vi "String to Control loop cluster.vi"(11 "Control Loop Details":string="EXCT:TYPE:Unipolar:MAG:10.00:EXCT:NICK:MB1.T1:LOOP:AUX:None:PSET:1.0:HTR:None:ISET:1.0:HAUT:Manual:HSET:0.0:PIDT:Manual:DSET:1.0:TSET:0K:LVL:MB1.T1:LOOP:MAN:HVER:0:FVER:20.6:SERL:102750119:MAN:CAL:OFFS:0.0000:COLD:1.0000:INT:Linear:SCAL:1.0000:FILE:RP5.DAT:HOTL:1023.1500:CAL:TYPE:PTC:SIG:VOLT:1405.9mV:CURR:10µA:TEMP:1023.15K:POWR:14.059µW:RES:140590?:SLOP:137.409?/K:FLOW:NOT_FOUND:SIG:TEMP\n") -> (3 "Control Loop":T1)   [LabVIEW 2015, in "Mercury iXX.lvlib" / "Control Loop.lvlib"]
uses:
  Control Loop.lvlib
  Temperature/Controls/Loop Cluster.ctl
  Temperature.lvlib
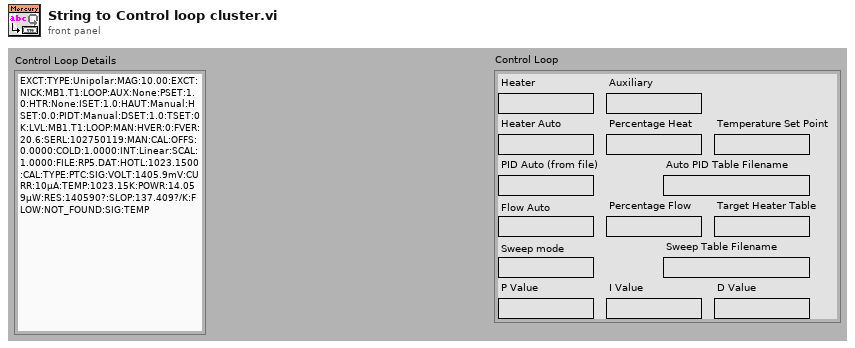
[diagram p1: front panel]
types:
  T1 = typedef "Mercury iXX.lvlib/Temperature.lvlib/Loop Cluster.ctl" = cluster{"Heater":string, "Auxiliary":string, "Heater Auto":string, "Percentage Heat":string, "Temperature Set Point":string, "PID Auto (from file)":string, "P Value":string, "I Value":string, "D Value":string, "Auto PID Table Filename":string, "Flow Auto":string, "Target Heater Table":string, "Sweep mode":string, "Sweep Table Filename":string, "Percentage Flow":string}
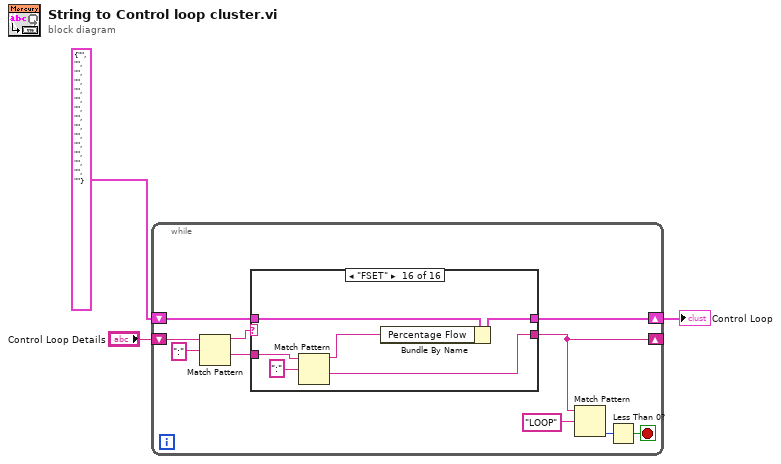
[diagram p0: block diagram]
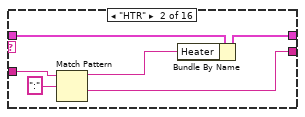
[diagram p3: hidden frame]
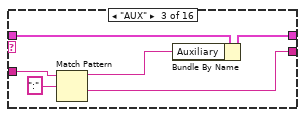
[diagram p4: hidden frame]
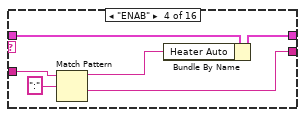
[diagram p5: hidden frame]
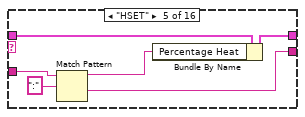
[diagram p6: hidden frame]
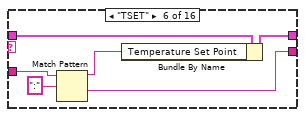
[diagram p7: hidden frame]
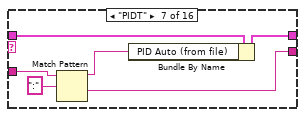
[diagram p8: hidden frame]
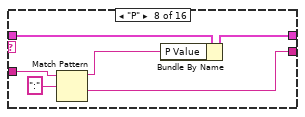
[diagram p9: hidden frame]
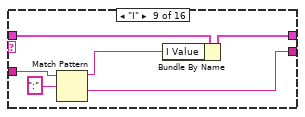
[diagram p10: hidden frame]
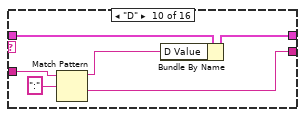
[diagram p11: hidden frame]
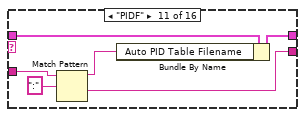
[diagram p12: hidden frame]
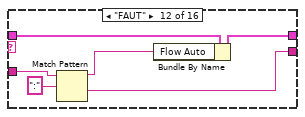
[diagram p13: hidden frame]
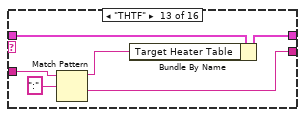
[diagram p14: hidden frame]
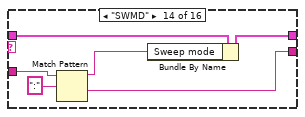
[diagram p15: hidden frame]
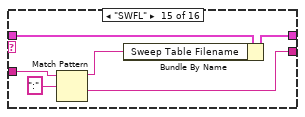
[diagram p16: hidden frame]
diagram:
  n1 = while {
    shift-right: [w6] -> w2
    shift-left: T1 {"Heater"="", "Auxiliary"="", "Heater Auto"="", "Percentage Heat"="", "Temperature Set Point"="", "PID Auto (from file)"="", "P Value"="", "I Value"="", "D Value"="", "Auto PID Table Filename"="", "Flow Auto"="", "Target Heater Table"="", "Sweep mode"="", "Sweep Table Filename"="", "Percentage Flow"=""} ("Control Loop") -> [w7]
    shift-right: [w4] -> _
    shift-left: "Control Loop Details" -> [w12]
    stop <- w9 stop-if-true
    n2 = Match Pattern(string=w12, regular expression=":") -> (before substring=w11:string, after substring=w5:string)  [unwired: 3 out]
    n3 = case shown="\"FSET\"" w11 {
      tunnel: w7 -> [w15 w17 w23 w29 w35 w41 w47 w53 w59 w65 w71 w77 w83 w89 w95 w101]
      tunnel: [w15 w18 w24 w30 w36 w42 w48 w54 w60 w66 w72 w78 w84 w90 w96 w102] -> w6
      tunnel: [w14 w19 w25 w31 w37 w43 w49 w55 w61 w67 w73 w79 w85 w91 w97 w103] -> w4
      tunnel: w5 -> [w14 w20 w26 w32 w38 w44 w50 w56 w62 w68 w74 w80 w86 w92 w98 w104]
      frame "", Default {
      }
      frame "HTR" {
        n4 = Match Pattern(string=w20, regular expression=":") -> (before substring=w16:string, after substring=w19:string)  [unwired: 3 out]
        n5 = Bundle By Name(cluster=w17, "Heater"=w16) -> (w18:T1)
      }
      frame "AUX" {
        n6 = Match Pattern(string=w26, regular expression=":") -> (before substring=w22:string, after substring=w25:string)  [unwired: 3 out]
        n7 = Bundle By Name(cluster=w23, "Auxiliary"=w22) -> (w24:T1)
      }
      frame "ENAB" {
        n8 = Match Pattern(string=w32, regular expression=":") -> (before substring=w28:string, after substring=w31:string)  [unwired: 3 out]
        n9 = Bundle By Name(cluster=w29, "Heater Auto"=w28) -> (w30:T1)
      }
      frame "HSET" {
        n10 = Match Pattern(string=w38, regular expression=":") -> (before substring=w34:string, after substring=w37:string)  [unwired: 3 out]
        n11 = Bundle By Name(cluster=w35, "Percentage Heat"=w34) -> (w36:T1)
      }
      frame "TSET" {
        n12 = Match Pattern(string=w44, regular expression=":") -> (before substring=w40:string, after substring=w43:string)  [unwired: 3 out]
        n13 = Bundle By Name(cluster=w41, "Temperature Set Point"=w40) -> (w42:T1)
      }
      frame "PIDT" {
        n14 = Match Pattern(string=w50, regular expression=":") -> (before substring=w46:string, after substring=w49:string)  [unwired: 3 out]
        n15 = Bundle By Name(cluster=w47, "PID Auto (from file)"=w46) -> (w48:T1)
      }
      frame "P" {
        n16 = Match Pattern(string=w56, regular expression=":") -> (before substring=w52:string, after substring=w55:string)  [unwired: 3 out]
        n17 = Bundle By Name(cluster=w53, "P Value"=w52) -> (w54:T1)
      }
      frame "I" {
        n18 = Match Pattern(string=w62, regular expression=":") -> (before substring=w58:string, after substring=w61:string)  [unwired: 3 out]
        n19 = Bundle By Name(cluster=w59, "I Value"=w58) -> (w60:T1)
      }
      frame "D" {
        n20 = Match Pattern(string=w68, regular expression=":") -> (before substring=w64:string, after substring=w67:string)  [unwired: 3 out]
        n21 = Bundle By Name(cluster=w65, "D Value"=w64) -> (w66:T1)
      }
      frame "PIDF" {
        n22 = Match Pattern(string=w74, regular expression=":") -> (before substring=w70:string, after substring=w73:string)  [unwired: 3 out]
        n23 = Bundle By Name(cluster=w71, "Auto PID Table Filename"=w70) -> (w72:T1)
      }
      frame "FAUT" {
        n24 = Match Pattern(string=w80, regular expression=":") -> (before substring=w76:string, after substring=w79:string)  [unwired: 3 out]
        n25 = Bundle By Name(cluster=w77, "Flow Auto"=w76) -> (w78:T1)
      }
      frame "THTF" {
        n26 = Match Pattern(string=w86, regular expression=":") -> (before substring=w82:string, after substring=w85:string)  [unwired: 3 out]
        n27 = Bundle By Name(cluster=w83, "Target Heater Table"=w82) -> (w84:T1)
      }
      frame "SWMD" {
        n28 = Match Pattern(string=w92, regular expression=":") -> (before substring=w88:string, after substring=w91:string)  [unwired: 3 out]
        n29 = Bundle By Name(cluster=w89, "Sweep mode"=w88) -> (w90:T1)
      }
      frame "SWFL" {
        n30 = Match Pattern(string=w98, regular expression=":") -> (before substring=w94:string, after substring=w97:string)  [unwired: 3 out]
        n31 = Bundle By Name(cluster=w95, "Sweep Table Filename"=w94) -> (w96:T1)
      }
      frame "FSET" {
        n32 = Match Pattern(string=w104, regular expression=":") -> (before substring=w100:string, after substring=w103:string)  [unwired: 3 out]
        n33 = Bundle By Name(cluster=w101, "Percentage Flow"=w100) -> (w102:T1)
      }
    }
    n34 = Match Pattern(string=w4, regular expression="LOOP") -> (offset past match=w10:i32)  [unwired: 4 out]
    n35 = Less Than 0?(x=w10) -> (x < 0?=w9:bool)
  }
  "Control Loop" <- w2
